vi "BRig_dataCurrent_t_selection.vi"() -> (2 "output_t_selection":i32)   [LabVIEW 2014]
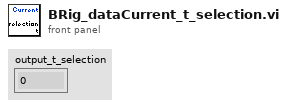
[diagram p1: front panel]
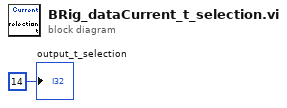
[diagram p0: block diagram]
diagram:
  "output_t_selection" <- 14 ("output_iBlock")
